vi "Read Module.vi"(8 "error in (no error)":errorcluster, 11 "Write to Module Msg in":refnum<class "Write to Module Msg.lvclass">) -> (0 "error out":errorcluster, 2 "Module":enum16{"LAI", "LDO", "Control"}(ring), 3 "Write to Module Msg out":refnum<class "Write to Module Msg.lvclass">)   [LabVIEW 2020, in "Modbus.lvlib" / "Write to Module Msg.lvclass"]
uses:
  Write to Module Msg.lvclass
  Write to Module Msg.lvclass/Write to Module Msg.ctl
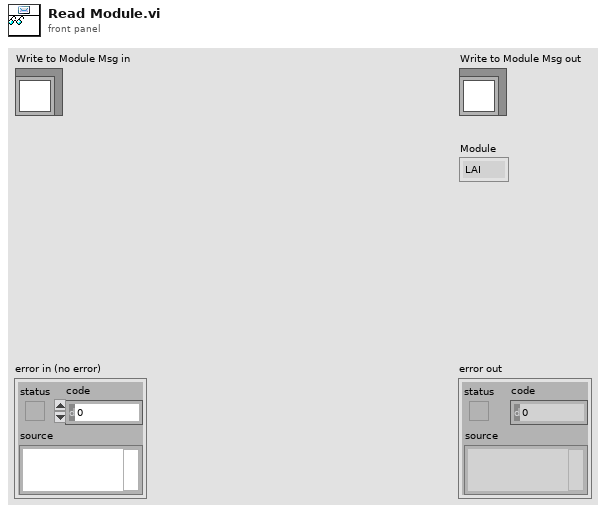
[diagram p1: front panel]
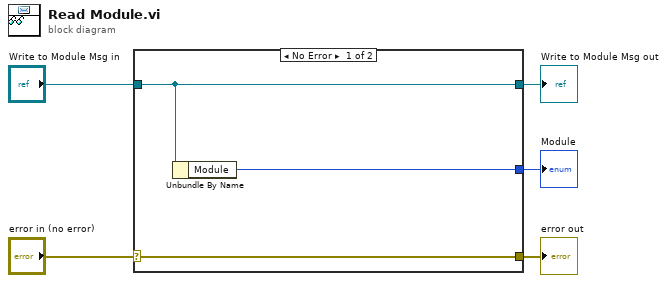
[diagram p0: block diagram]
diagram:
  n1 = case shown="No Error" "error in (no error)" {
    selector: "error in (no error)" -> [w8 w9]
    tunnel: [w8 w9] -> w4
    tunnel: [w7 w10] -> w2
    tunnel: "Write to Module Msg in" -> [w7 w10]
    tunnel: [w6 _] -> w1
    frame No Error {
      n2 = Unbundle By Name(w7) -> ("Module"=w6:enum16{"LAI", "LDO", "Control"})
    }
    frame Error {
    }
  }
  "error out" <- w4
  "Write to Module Msg out" <- w2
  "Module" <- w1
